vi "Queue Comms EnQueue.vi"(8 "error in":errorcluster, 10 "Module Data Cluster":T1) -> (0 "error out":errorcluster)   [LabVIEW 2018, in "Entry Console.lvlib"]
uses:
  Entry Console.lvlib
  Private Controls/Module Data Cluster.ctl
  Private Controls/Module Action.ctl
  Private Controls/Queue FG Action.ctl
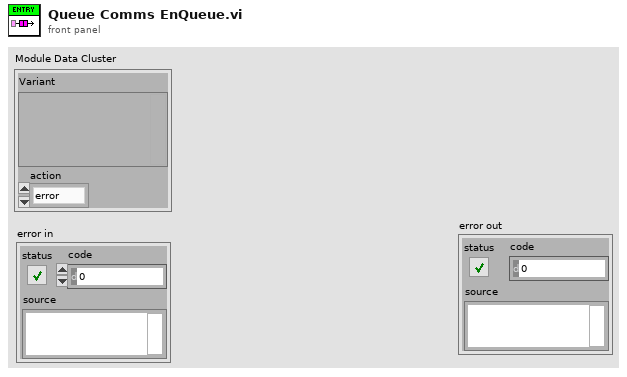
[diagram p1: front panel]
types:
  T1 = typedef "Entry Console.lvlib/Module Data Cluster.ctl" = cluster{"Variant":variant, "action":T2}
  T2 = typedef "Entry Console.lvlib/Module Action.ctl" = enum16{"error", "exit", "Start Wash", "init", "Enable Wash Buttons"}
  T3 = typedef "Entry Console.lvlib/Queue FG Action.ctl" = enum16{"Release", "Get", "Set"}
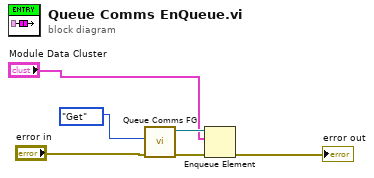
[diagram p0: block diagram]
diagram:
  n1 = call "Queue Comms FG.vi"("error in"="error in", "Action"=Queue_FG_Action."Get") -> ("error out"=w5:errorcluster, "queue out"=w4:refnum<queue>)  [unwired: 8 in]
  n2 = Enqueue Element(queue=w4, element="Module Data Cluster", error in (no error)=w5) -> (error out=→"error out":errorcluster)  [unwired: 1 in, 2 out]
